vi "CANOpen_NMT_Read HW Inputs.vi"(8 "error in":errorcluster, 10 "Hardware Input FIFO":refnum<k33>, 11 "Channel Pairs":T1 {"Chan Refs" format="%.0x"}) -> (0 "error out":errorcluster, 2 "Read Occured":bool, 3 "Channel Pairs Out":T1 {"Chan Refs" format="%.0x"})   [LabVIEW 2013, in "CANOpen Addon Custom Device.lvlib"]
uses:
  CANOpen Addon Custom Device.lvlib
  CanOpen_NMT_HWIn_ChannelPairs.ctl
  <vilib>/NI Veristand/Custom Device API/Data Reference.ctl
  <vilib>/NI Veristand/Custom Device API/Global Data Refs.vi
  <vilib>/NI Veristand/Custom Device API/Custom Device API.lvlib
  Debug/SubVIs/Global debug.vi
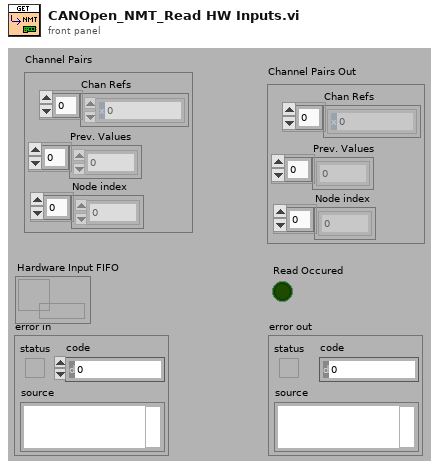
[diagram p1: front panel]
types:
  T1 = typedef "CANOpen Addon Custom Device.lvlib/CanOpen_NMT_HWIn_ChannelPairs.ctl" = cluster{"Chan Refs":T2[], "Prev. Values":dbl[], "Node index":dbl[]}
  T2 = typedef "Custom Device API.lvlib/Data Reference.ctl" = i32
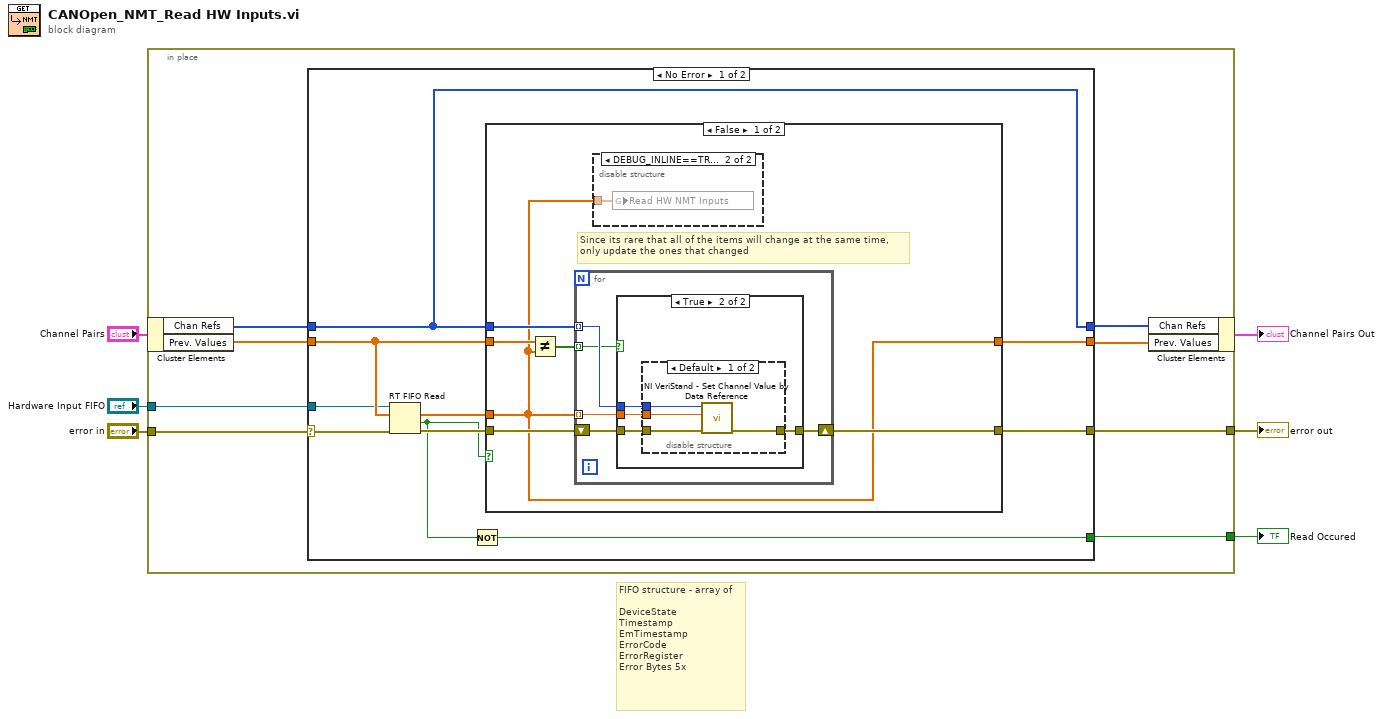
[diagram p0: block diagram]
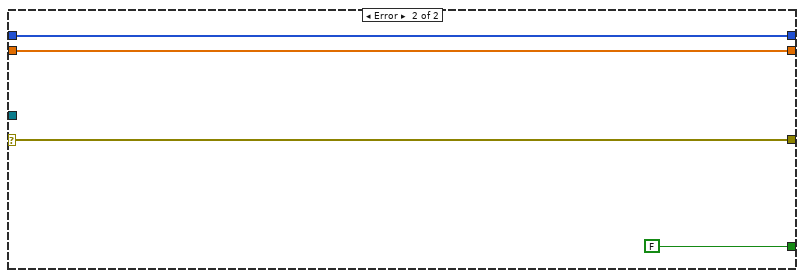
[diagram p6: hidden frame]
diagram:
  # "FIFO structure - array of\n\nDeviceState\nTimestamp\nEmTimestamp\nErrorCode\nErrorRegister\nError Bytes 5x"
  n1 = in-place {
    in-place-border: [w14] -> w6
    in-place-border: [w13] -> w5
    in-place-border: "error in" -> [w8]
    in-place-border: "Hardware Input FIFO" -> [w7]
    n2 = in-place-cluster #1("Channel Pairs") -> ("Chan Refs"=w12:T2[], "Prev. Values"=w11:dbl[])
    n3 = case shown="No Error" w8 {
      selector: w8 -> [w21 w52]
      tunnel: [w24 w52] -> w14
      tunnel: [w17 w50] -> w10
      tunnel: [w19 FALSE ("C Read Occured?")] -> w13
      tunnel: w12 -> [w16 w49]
      tunnel: w11 -> [w18 w50]
      tunnel: [w16 w49] -> w9
      tunnel: w7 -> [w15 _]
      frame No Error {
        n4 = RT FIFO Read(0:w15, 1:w18, 3:w21) -> (9:w22:dbl[], 10:w20:bool, 11:w23:errorcluster)  [unwired: 1 in, 2 out]
        n5 = Not(x=w20) -> (.not. x?=w19:bool)
        n6 = case shown="False" w20 {
          tunnel: w23 -> [w30 w48]
          tunnel: w22 -> [w25 _]
          tunnel: [w29 w48] -> w24
          tunnel: [w25 w47] -> w17
          tunnel: w16 -> [w28 _]
          tunnel: w18 -> [w26 w47]
          frame False {
            # "Since its rare that all of the items will change at the same time,\nonly update the ones that changed"
            n7 = Not Equal?(x=w26, y=w25) -> (x != y?=w27:bool[])
            n8 = for {
              shift-right: [w36] -> w29
              shift-left: w30 -> [w35]
              tunnel: w27 -> [w33] mode=indexing
              tunnel: w25 -> [w32] mode=indexing
              tunnel: w28 -> [w34] mode=indexing
              n9 = case shown="True" w33 {
                tunnel: w32 -> [_ w38]
                tunnel: [w37 w40] -> w36
                tunnel: w35 -> [w37 w41]
                tunnel: w34 -> [_ w39]
                frame False {
                }
                frame True {
                  n10 = disable-structure shown="Default" {
                    disable-tunnel: w41 -> [w45 w46]
                    disable-tunnel: [w44 w46] -> w40
                    disable-tunnel: w39 -> [w43 _]
                    disable-tunnel: w38 -> [w42 _]
                    frame condition #0 (active) {
                      n11 = call <vilib>:"NI VeriStand - Set Channel Value by Data Reference.vi"("error in (no error)"=w45, "Value"=w42, "Data Reference in"=w43) -> ("error out"=w44:errorcluster)  [unwired: 8 in]
                    }
                    frame condition #1 {
                    }
                  }
                }
              }
            }
            n12 = disable-structure shown="DEBUG_INLINE==TRUE" {
              disable-tunnel: w25 -> [_ w31]
              frame condition #0 (active) {
              }
              frame condition #1 {
                n13 = global write "Global debug.vi" "Read HW NMT Inputs"(w31) -> ()
              }
            }
          }
          frame True {
          }
        }
      }
      frame Error {
      }
    }
    n14 = in-place-cluster #1("Chan Refs"=w9, "Prev. Values"=w10) -> (→"Channel Pairs Out":T1)
  }
  "error out" <- w6
  "Read Occured" <- w5
